vi "Set Zone Indicators Color.vi"(8 "error in":errorcluster, 10 "Alert Status":T1, 11 "reference":refnum<vi>) -> (0 "error out":errorcluster)   [LabVIEW 2016]
doc: "Selects LED indicator color based on the status received."
uses:
  Controls/Zones Condition.ctl
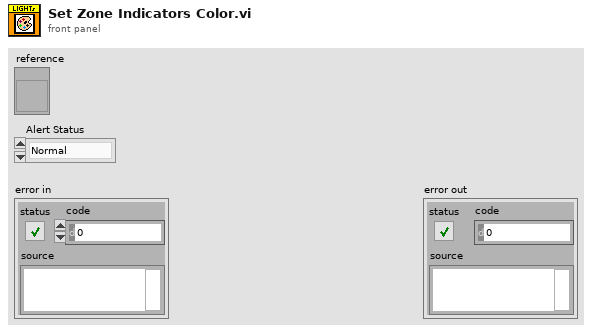
[diagram p1: front panel]
types:
  T1 = typedef "Zones Condition.ctl" = enum16{"Normal", "Bypass", "Tamper", "Alarm"}
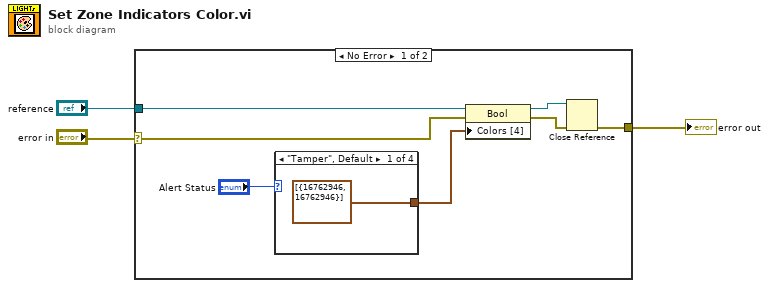
[diagram p0: block diagram]
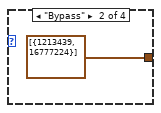
[diagram p2: hidden frame]
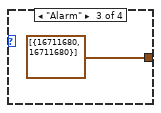
[diagram p3: hidden frame]
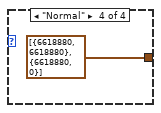
[diagram p4: hidden frame]
diagram:
  n1 = case shown="No Error" "error in" {
    selector: "error in" -> [w10 w15]
    tunnel: [w4 w15] -> w2
    tunnel: "reference" -> [w6 _]
    frame No Error {
      n2 = case shown="\"Tamper\", Default" "Alert Status" {
        tunnel: [cluster{"Color Box":u32, "Color Box":u32}[] [{"Color Box"=16762946, "Color Box"=16762946}] ("Colors [4]") cluster{"Color Box":u32, "Color Box":u32}[] [{"Color Box"=1213439, "Color Box"=16777224}] ("Colors [4]") cluster{"Color Box":u32, "Color Box":u32}[] [{"Color Box"=16711680, "Color Box"=16711680}] ("Colors [4]") cluster{"Color Box":u32, "Color Box":u32}[] [{"Color Box"=6618880, "Color Box"=6618880}, {"Color Box"=6618880, "Color Box"=0}] ("Colors [4]")] -> w9
        frame "Tamper", Default {
        }
        frame "Bypass" {
        }
        frame "Alarm" {
        }
        frame "Normal" {
        }
      }
      n3 = property class="Bool"(reference=w6, error in=w10, "Colors [4]"=w9) -> (reference out=w7:refnum<vi>, error out=w8:errorcluster)
      n4 = Close Reference(reference=w7, error in (no error)=w8) -> (error out=w4:errorcluster)
    }
    frame Error {
    }
  }
  "error out" <- w2
